vi "PlsGen_Angle_Convert.vi"(0 "TDC (Absolute CAD)":sgl, 1 "MaxCAD":sgl, 2 "FPGA Clock Frequency (MHz, 40)":sgl=40.0 format="%#_6f", 5 "Channel Enable":bool, 7 "PlsGen_Angle_Config_In":T2) -> (8 "PlsGen_Config_Out":T1)   [LabVIEW 2015, in "ECS-RT.lvlib"]
doc: "This VI is used to convert a sequence of up to five angle-based injection pulses to FPGA-based clock ticks and Crank Angle Ticks (CAT) for each channel of the DI Driver module. The PlsGen_config cluster is configured for an overall window of operation, individual pulse enabling, injection pulse start-angle, and pulse duration. The operating windows for each channel must not overlap."
uses:
  ECS-RT.lvlib
  Typedefs/Raw Outputs/DI.ctl
  <vilib>/Powertrain Controls/Device Drivers/Engine Position Tracking/EPTx/RevA/RT/EPTx - RevA - RT.lvlib
  ECS-Shared.lvlib
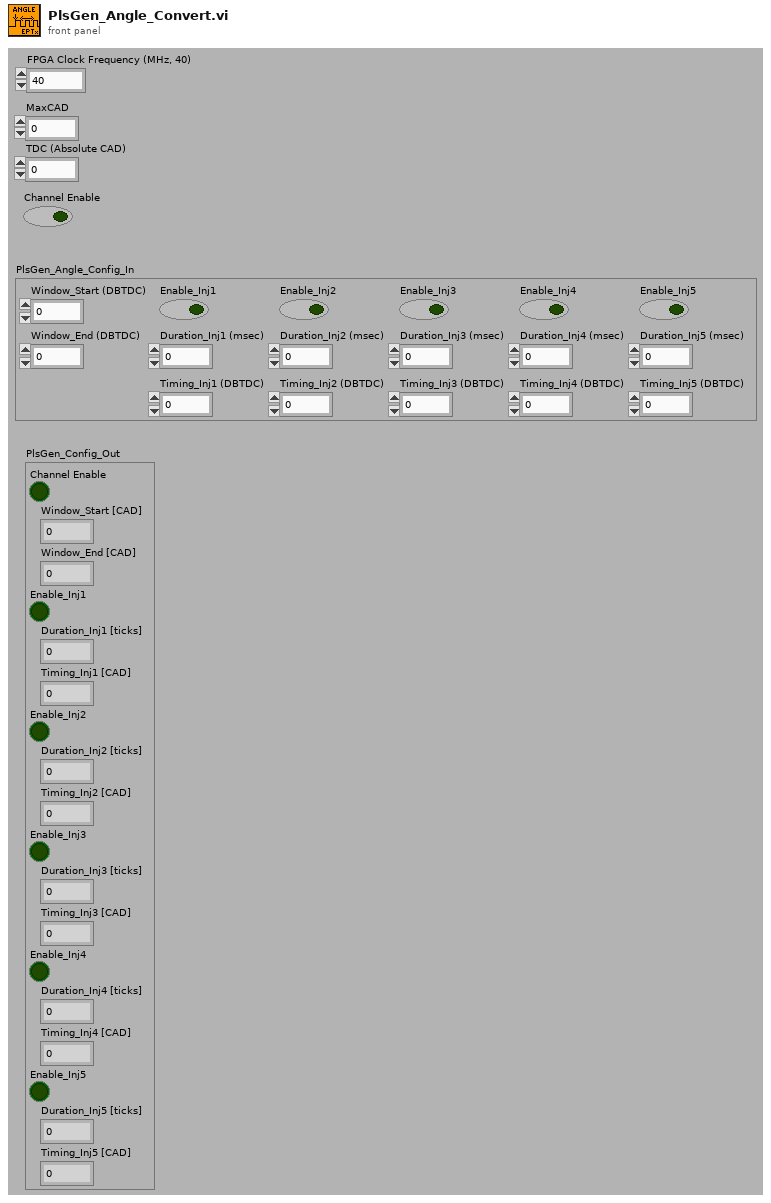
[diagram p1: front panel]
types:
  T1 = cluster{"Channel Enable":bool, "Window_Start [CAD]":fxp<+,18,11>, "Window_End [CAD]":fxp<+,18,11>, "Enable_Inj1":bool, "Duration_Inj1 [ticks]":u32, "Timing_Inj1 [CAD]":fxp<+,18,11>, "Enable_Inj2":bool, "Duration_Inj2 [ticks]":u32, "Timing_Inj2 [CAD]":fxp<+,18,11>, "Enable_Inj3":bool, "Duration_Inj3 [ticks]":u32, "Timing_Inj3 [CAD]":fxp<+,18,11>, "Enable_Inj4":bool, "Duration_Inj4 [ticks]":u32, "Timing_Inj4 [CAD]":fxp<+,18,11>, "Enable_Inj5":bool, "Duration_Inj5 [ticks]":u32, "Timing_Inj5 [CAD]":fxp<+,18,11>}
  T2 = typedef "ECS-Shared.lvlib/DI.ctl" = cluster{"Window_Start (DBTDC)":sgl, "Window_End (DBTDC)":sgl, "Enable_Inj1":bool, "Duration_Inj1 (msec)":sgl, "Timing_Inj1 (DBTDC)":sgl, "Enable_Inj2":bool, "Duration_Inj2 (msec)":sgl, "Timing_Inj2 (DBTDC)":sgl, "Enable_Inj3":bool, "Duration_Inj3 (msec)":sgl, "Timing_Inj3 (DBTDC)":sgl, "Enable_Inj4":bool, "Duration_Inj4 (msec)":sgl, "Timing_Inj4 (DBTDC)":sgl, "Enable_Inj5":bool, "Duration_Inj5 (msec)":sgl, "Timing_Inj5 (DBTDC)":sgl}
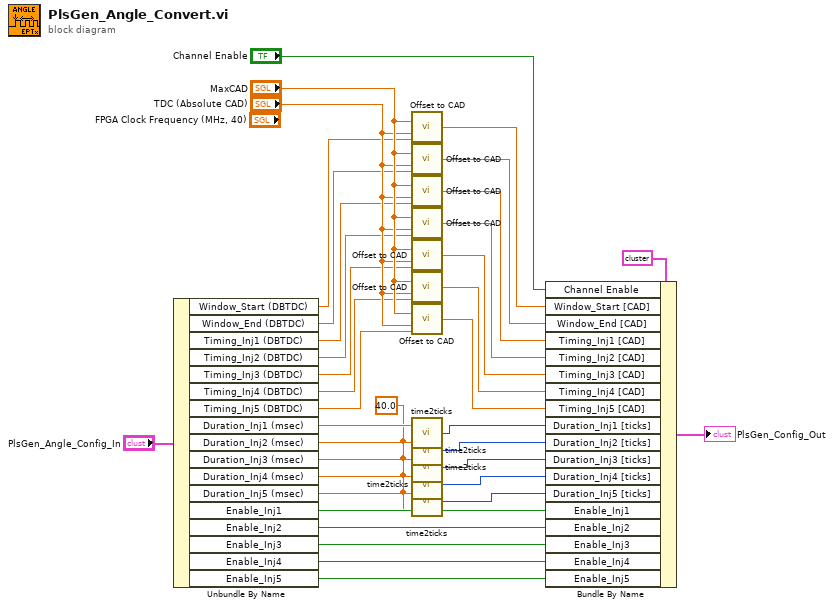
[diagram p0: block diagram]
diagram:
  w2 = sgl 40.0 ("Clock Frequency (MHz, 40)")
  n1 = Unbundle By Name("PlsGen_Angle_Config_In") -> ("Window_Start (DBTDC)"=w26:sgl, "Window_End (DBTDC)"=w25:sgl, "Timing_Inj1 (DBTDC)"=w20:sgl, "Timing_Inj2 (DBTDC)"=w21:sgl, "Timing_Inj3 (DBTDC)"=w22:sgl, "Timing_Inj4 (DBTDC)"=w23:sgl, "Timing_Inj5 (DBTDC)"=w24:sgl, "Duration_Inj1 (msec)"=w12:sgl, "Duration_Inj2 (msec)"=w10:sgl, "Duration_Inj3 (msec)"=w9:sgl, "Duration_Inj4 (msec)"=w8:sgl, "Duration_Inj5 (msec)"=w11:sgl, "Enable_Inj1"=w27:bool, "Enable_Inj2"=w28:bool, "Enable_Inj3"=w33:bool, "Enable_Inj4"=w29:bool, "Enable_Inj5"=w30:bool)
  n2 = call <vilib>:"Offset to CAD.vi"("Max CAD"="MaxCAD", "Cylinder TDC [Absolute CAD]"="TDC (Absolute CAD)", "Offset [DBTDC]"=w26) -> ("CAD [Absolute CAD]"=w31:sgl)  [unwired: 12 in]
  n3 = call <vilib>:"Offset to CAD.vi"("Max CAD"="MaxCAD", "Cylinder TDC [Absolute CAD]"="TDC (Absolute CAD)", "Offset [DBTDC]"=w25) -> ("CAD [Absolute CAD]"=w32:sgl)  [unwired: 12 in]
  n4 = call <vilib>:"Offset to CAD.vi"("Max CAD"="MaxCAD", "Cylinder TDC [Absolute CAD]"="TDC (Absolute CAD)", "Offset [DBTDC]"=w20) -> ("CAD [Absolute CAD]"=w15:sgl)  [unwired: 12 in]
  n5 = call <vilib>:"Offset to CAD.vi"("Max CAD"="MaxCAD", "Cylinder TDC [Absolute CAD]"="TDC (Absolute CAD)", "Offset [DBTDC]"=w21) -> ("CAD [Absolute CAD]"=w16:sgl)  [unwired: 12 in]
  n6 = call <vilib>:"Offset to CAD.vi"("Max CAD"="MaxCAD", "Cylinder TDC [Absolute CAD]"="TDC (Absolute CAD)", "Offset [DBTDC]"=w22) -> ("CAD [Absolute CAD]"=w17:sgl)  [unwired: 12 in]
  n7 = call <vilib>:"Offset to CAD.vi"("Max CAD"="MaxCAD", "Cylinder TDC [Absolute CAD]"="TDC (Absolute CAD)", "Offset [DBTDC]"=w23) -> ("CAD [Absolute CAD]"=w18:sgl)  [unwired: 12 in]
  n8 = call <vilib>:"Offset to CAD.vi"("Max CAD"="MaxCAD", "Cylinder TDC [Absolute CAD]"="TDC (Absolute CAD)", "Offset [DBTDC]"=w24) -> ("CAD [Absolute CAD]"=w19:sgl)  [unwired: 12 in]
  n9 = call <vilib>:"time2ticks.vi"("Clock Frequency (MHz, 40)"=w2, "Time (msec)"=w12) -> ("Ticks"=w7:u32)
  n10 = call <vilib>:"time2ticks.vi"("Clock Frequency (MHz, 40)"=w2, "Time (msec)"=w10) -> ("Ticks"=w6:u32)
  n11 = call <vilib>:"time2ticks.vi"("Clock Frequency (MHz, 40)"=w2, "Time (msec)"=w9) -> ("Ticks"=w5:u32)
  n12 = call <vilib>:"time2ticks.vi"("Clock Frequency (MHz, 40)"=w2, "Time (msec)"=w8) -> ("Ticks"=w4:u32)
  n13 = call <vilib>:"time2ticks.vi"("Clock Frequency (MHz, 40)"=w2, "Time (msec)"=w11) -> ("Ticks"=w3:u32)
  n14 = Bundle By Name(cluster=T1 {"Channel Enable"=FALSE, "Window_Start [CAD]"=0.0, "Window_End [CAD]"=0.0, "Enable_Inj1"=FALSE, "Duration_Inj1 [ticks]"=0, "Timing_Inj1 [CAD]"=0.0, "Enable_Inj2"=FALSE, "Duration_Inj2 [ticks]"=0, "Timing_Inj2 [CAD]"=0.0, "Enable_Inj3"=FALSE, "Duration_Inj3 [ticks]"=0, "Timing_Inj3 [CAD]"=0.0, "Enable_Inj4"=FALSE, "Duration_Inj4 [ticks]"=0, "Timing_Inj4 [CAD]"=0.0, "Enable_Inj5"=FALSE, "Duration_Inj5 [ticks]"=0, "Timing_Inj5 [CAD]"=0.0} ("DI-1.PlsGen_Config_Channel3"), "Channel Enable"="Channel Enable", "Window_Start [CAD]"=w31, "Window_End [CAD]"=w32, "Timing_Inj1 [CAD]"=w15, "Timing_Inj2 [CAD]"=w16, "Timing_Inj3 [CAD]"=w17, "Timing_Inj4 [CAD]"=w18, "Timing_Inj5 [CAD]"=w19, "Duration_Inj1 [ticks]"=w7, "Duration_Inj2 [ticks]"=w6, "Duration_Inj3 [ticks]"=w5, "Duration_Inj4 [ticks]"=w4, "Duration_Inj5 [ticks]"=w3, "Enable_Inj1"=w27, "Enable_Inj2"=w28, "Enable_Inj3"=w33, "Enable_Inj4"=w29, "Enable_Inj5"=w30) -> (→"PlsGen_Config_Out":T1)
